vi "Get Age.vi"(8 "error in (no error)":errorcluster, 11 "Person in":refnum<class "Person.lvclass">) -> (0 "error out":errorcluster, 2 "Age":i32, 3 "Person out":refnum<class "Person.lvclass">)   [LabVIEW 2017, in "Person.lvclass"]
uses:
  Person.lvclass
  Person.lvclass/Person.ctl
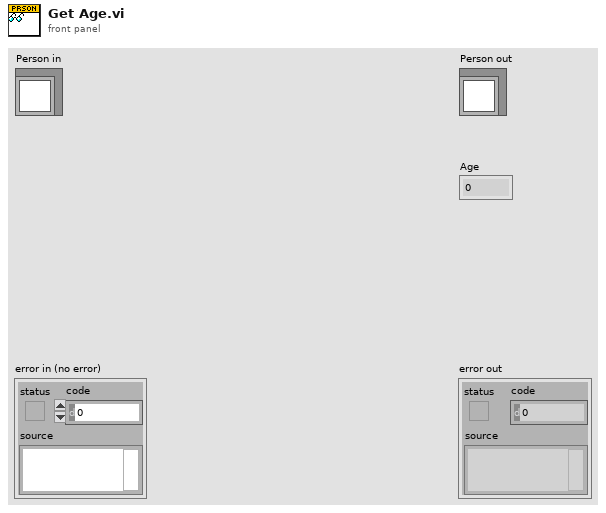
[diagram p1: front panel]
types:
  T1 = typedef "LVDateTimeRec.ctl" = cluster{"fractional second":dbl, "second":i32, "minute":i32, "hour":i32, "day of month":i32, "month":i32, "year":i32, "day of week":i32, "day of year":i32, "DST":i32}
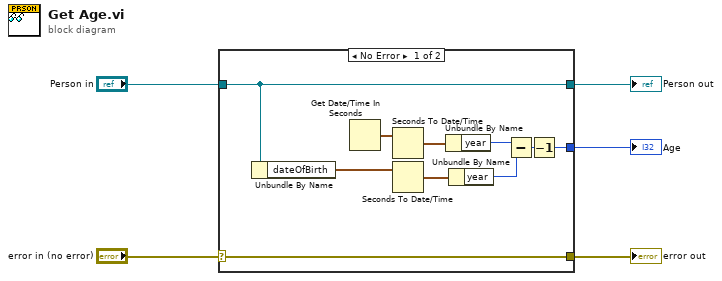
[diagram p0: block diagram]
diagram:
  n1 = case shown="No Error" "error in (no error)" {
    selector: "error in (no error)" -> [w15 w16]
    tunnel: [w15 w16] -> w4
    tunnel: [w14 w17] -> w2
    tunnel: "Person in" -> [w14 w17]
    tunnel: [w6 _] -> w1
    frame No Error {
      n2 = Unbundle By Name(w14) -> ("dateOfBirth"=w7:timestamp)
      n3 = Get Date/Time In Seconds() -> (seconds since 1Jan1904=w13:timestamp)
      n4 = Seconds To Date/Time(time stamp (now)=w13) -> (date time rec=w11:T1)  [unwired: 1 in]
      n5 = Seconds To Date/Time(time stamp (now)=w7) -> (date time rec=w10:T1)  [unwired: 1 in]
      n6 = Unbundle By Name(w11) -> ("year"=w9:i32)
      n7 = Unbundle By Name(w10) -> ("year"=w8:i32)
      n8 = Subtract(x=w9, y=w8) -> (x-y=w12:i32)
      n9 = Decrement(x=w12) -> (x-1=w6:i32)
    }
    frame Error {
    }
  }
  "error out" <- w4
  "Person out" <- w2
  "Age" <- w1
